vi "master_filenames.vi"() -> ()   [LabVIEW 2017]
uses:
  <vilib>/Utility/file.llb/Write Delimited Spreadsheet (DBL).vi
  <vilib>/Utility/file.llb/Write Delimited Spreadsheet (string).vi
panel:
  out "Detected Voltage":string
  in  "VISA resource name":refnum<visa-resource-name>
  in  "file path (dialog if empty)":path
  out "Returned Y string":string
  out "Returned X string":string
  out "Incident Voltage":string
  in  "Number of Columns":i32
  out "data":dynamicdata(graph)
  in  "Number of Rows":i32
  in  "Sampling Rate (Hz)":dbl=100.0
  in  "Number of Samples":i32=100
  in  "Pixel Size (mm)":string
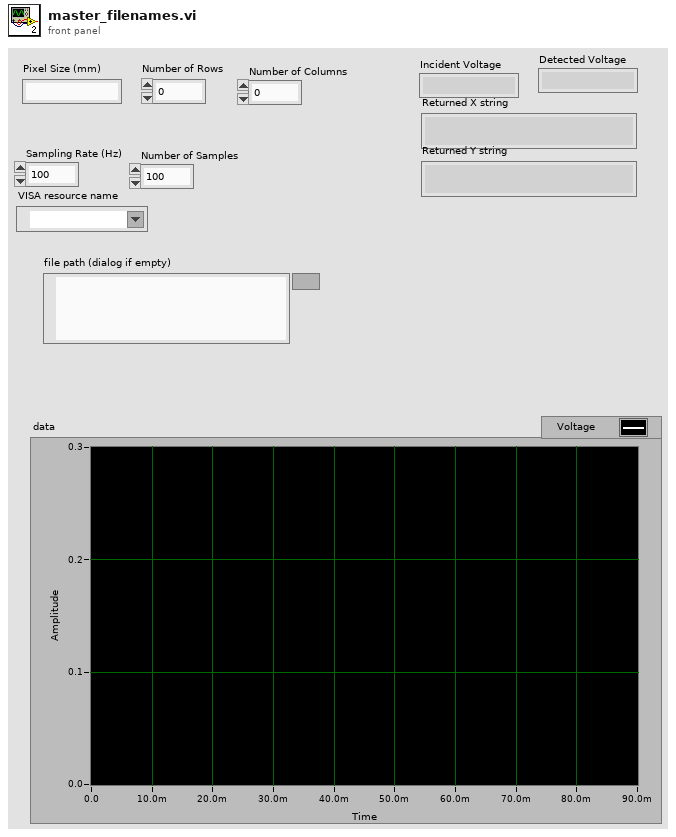
[diagram p1: front panel]
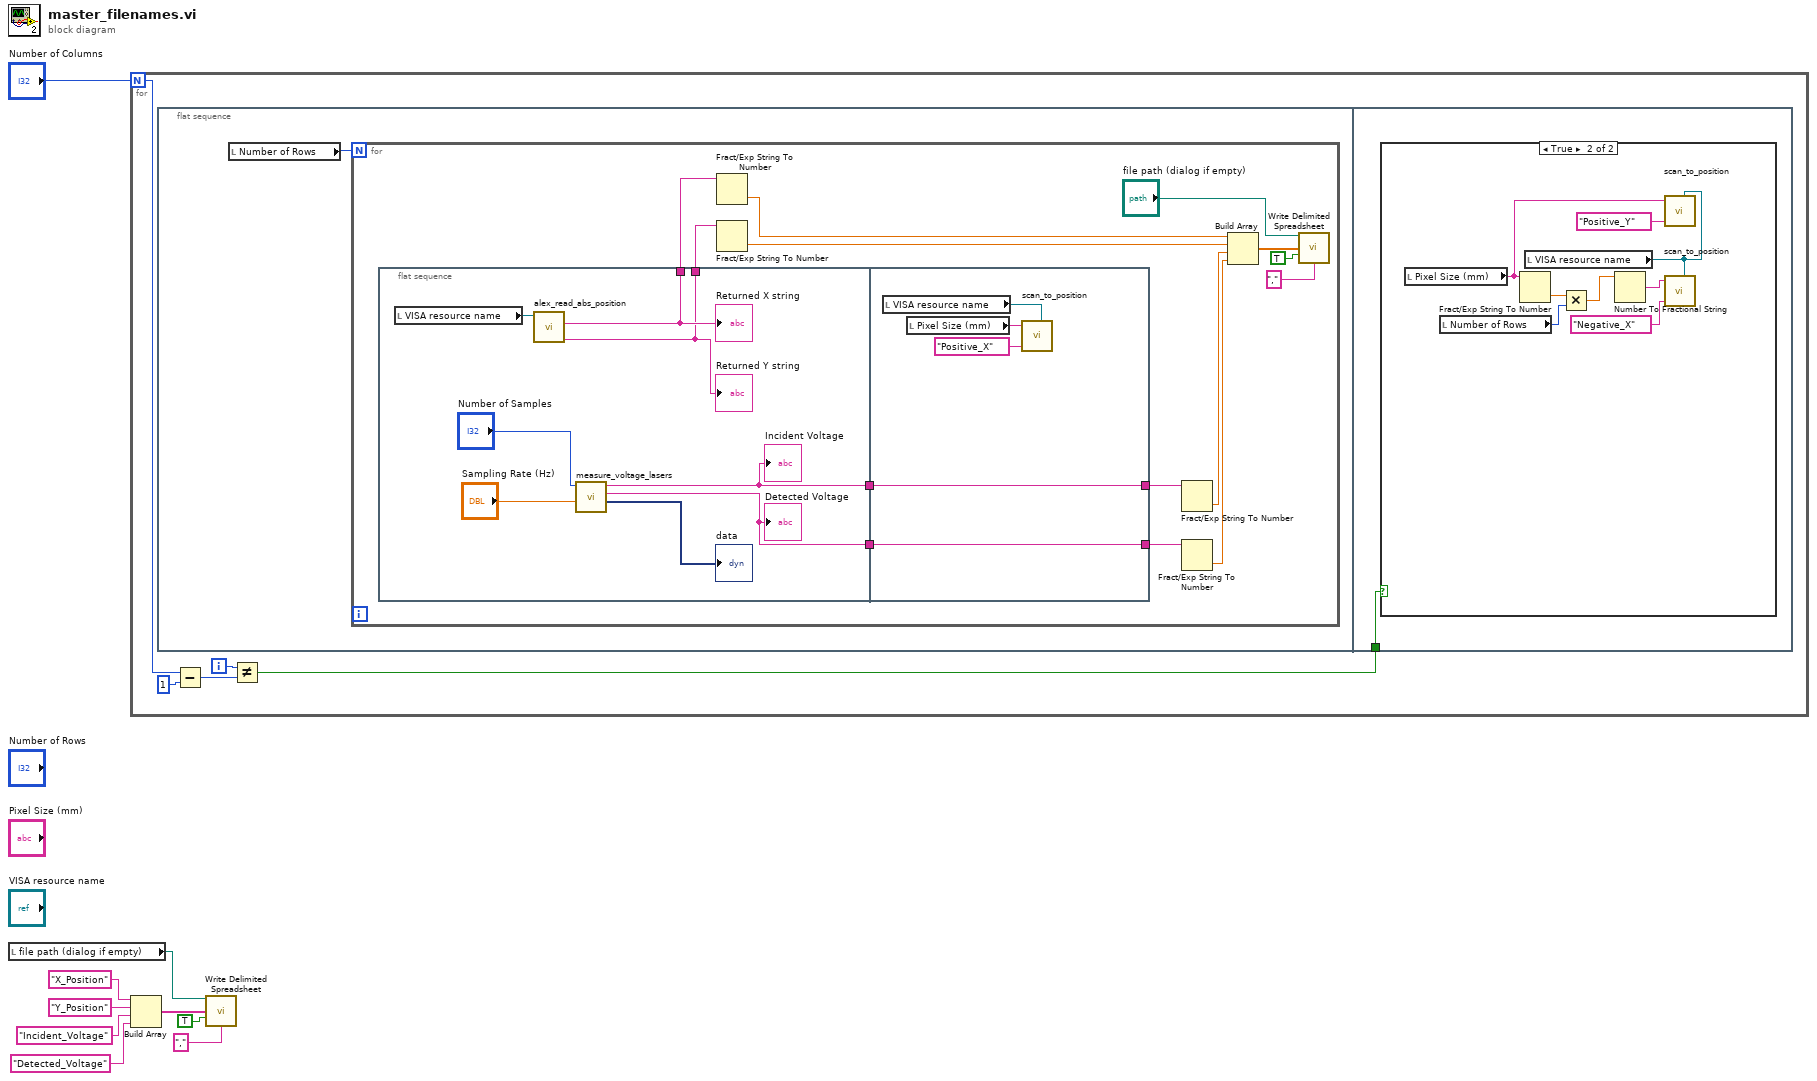
[diagram p0: block diagram]
diagram:
  n1 = local read "file path (dialog if empty)"() -> (w8:path)
  n2 = for {
    N: "Number of Columns" -> [w11]
    i -> [w12]
    n3 = flat-sequence {
      tunnel: w10 -> [w43]
      frame #0 {
        n4 = local read "Number of Rows"() -> (w15:i32)
        n5 = for {
          N: w15 -> [_]
          n6 = flat-sequence {
            tunnel: [w31] -> w21
            tunnel: [w37] -> w20
            tunnel: [w36] -> w19
            tunnel: [w30] -> w17
            tunnel: [w42] -> w27
            tunnel: w21 -> [w42]
            tunnel: [w38] -> w18
            tunnel: w17 -> [w38]
            frame #0 {
              n7 = local read "VISA resource name"() -> (w35:refnum<visa-resource-name>)
              n8 = call "alex_read_abs_position.vi"("VISA resource name"=w35) -> ("Returned Y string"=w36:string, "Returned X string"=w37:string)  [unwired: 9 in]
              "Returned X string" <- w37
              "Returned Y string" <- w36
              n9 = call "measure_voltage_lasers.vi"("rate"="Sampling Rate (Hz)", "number of samples"="Number of Samples") -> ("data"=→"data":dynamicdata, "Detected Voltage"=w30:string, "Incident Voltage"=w31:string)  [unwired: 6 in]
              "Incident Voltage" <- w31
              "Detected Voltage" <- w30
            }
            frame #1 {
              n10 = local read "VISA resource name"() -> (w40:refnum<visa-resource-name>)
              n11 = local read "Pixel Size (mm)"() -> (w39:string)
              n12 = call "scan_to_position.vi"("VISA resource name"=w40, "Direction to Move"="Positive_X", "Pixel Size (mm)"=w39) -> ()  [unwired: 6 in]
            }
          }
          n13 = Fract/Exp String To Number(string=w20) -> (number=w29:dbl)  [unwired: 3 in, 1 out]
          n14 = Fract/Exp String To Number(string=w19) -> (number=w28:dbl)  [unwired: 3 in, 1 out]
          n15 = Fract/Exp String To Number(string=w27) -> (number=w26:dbl)  [unwired: 3 in, 1 out]
          n16 = Fract/Exp String To Number(string=w18) -> (number=w16:dbl)  [unwired: 3 in, 1 out]
          n17 = Build Array(w29, w28, w26, w16) -> (w25:dbl[])
          n18 = call-poly <vilib>:"Write Delimited Spreadsheet.vi"("file path (dialog if empty)"="file path (dialog if empty)", "1D data"=w25, "append to file? (new file:F)"=TRUE, "delimiter (\\t)"="," ("delimiter (\\t)")) -> ()  [unwired: 10 in, 2 out]
        }
      }
      frame #1 {
        n19 = case shown="True" w43 {
          frame False {
          }
          frame True {
            n20 = local read "Pixel Size (mm)"() -> (w45:string)
            n21 = local read "Number of Rows"() -> (w44:i32)
            n22 = Fract/Exp String To Number(string=w45) -> (number=w49:dbl)  [unwired: 3 in, 1 out]
            n23 = local read "VISA resource name"() -> (w46:refnum<visa-resource-name>)
            n24 = Multiply(x=w49, y=w44) -> (x*y=w47:dbl)
            n25 = Number To Fractional String(number=w47) -> (F-format string=w48:string)  [unwired: 3 in]
            n26 = call "scan_to_position.vi"("VISA resource name"=w46, "Direction to Move"="Positive_Y", "Pixel Size (mm)"=w45) -> ()  [unwired: 6 in]
            n27 = call "scan_to_position.vi"("VISA resource name"=w46, "Direction to Move"="Negative_X", "Pixel Size (mm)"=w48) -> ()  [unwired: 6 in]
          }
        }
      }
    }
    n28 = Subtract(x=w11, y=1) -> (x-y=w13:i32)
    n29 = Not Equal?(x=w12, y=w13) -> (x != y?=w10:bool)
  }
  n30 = Build Array("X_Position", "Y_Position", "Incident_Voltage", "Detected_Voltage" ("element")) -> (w5:string[])
  n31 = call-poly <vilib>:"Write Delimited Spreadsheet.vi"("file path (dialog if empty)"=w8, "1D data"=w5, "append to file? (new file:F)"=TRUE, "delimiter (\\t)"="," ("delimiter (\\t)")) -> ()  [unwired: 10 in, 2 out]
